vi "Scalar SV Count - type code Array.vi"(8 "Error In":errorcluster) -> (0 "Error Out":errorcluster)   [LabVIEW 2014]
doc: "This VI counts the number of scalar shared variables."
panel:
  in  "Type code Array":i32[](array[numeric])
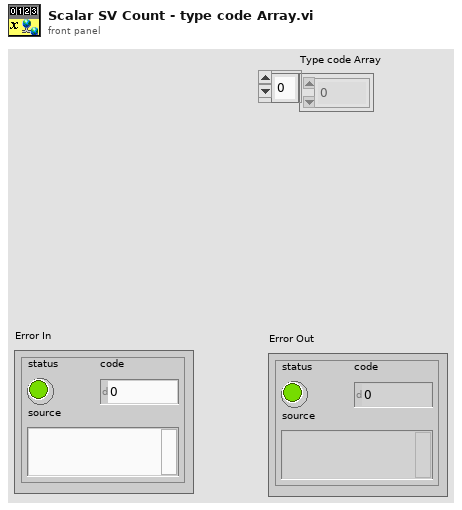
[diagram p1: front panel]
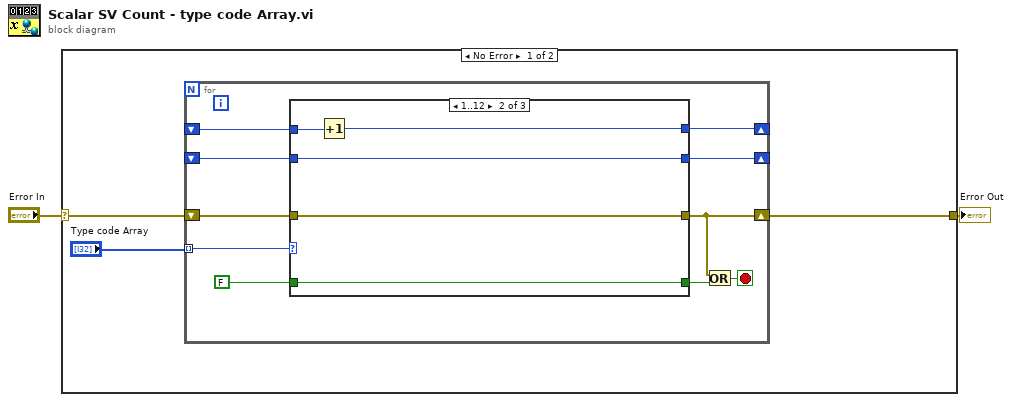
[diagram p0: block diagram]
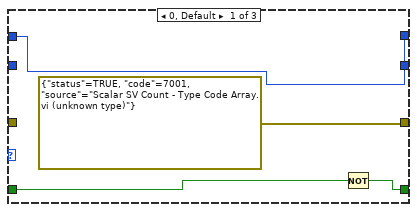
[diagram p2: hidden frame]
diagram:
  n1 = case shown="No Error" "Error In" {
    selector: "Error In" -> [w7 w30]
    tunnel: [w6 w30] -> w1
    frame No Error {
      n2 = for {
        shift-right: [w13] -> w6
        shift-left: w7 -> [w15]
        tunnel: "Type code Array" -> [w16] mode=indexing
        shift-right: [w10] -> _
        shift-left: [w12] -> w4
        shift-right: [w8] -> _
        shift-left: [w9] -> w3
        stop <- w14 stop-if-true
        n3 = case shown="1..12" w16 {
          tunnel: FALSE -> [w20 w23 w27]
          tunnel: w15 -> [_ w26 w29]
          tunnel: [errorcluster {"status"=TRUE, "code"=7001, "source"="Scalar SV Count - Type Code Array.vi (unknown type)"} ("error constant") w26 w29] -> w13
          tunnel: w12 -> [w18 w25 w28]
          tunnel: [w19 w23 w27] -> w11
          tunnel: [w18 w24 w28] -> w10
          tunnel: w9 -> [_ w22 _]
          tunnel: [_ w22 _] -> w8
          frame 0, Default {
            n4 = Not(x=w20) -> (.not. x?=w19:bool)
          }
          frame 1..12 {
            n5 = Increment(x=w25) -> (x+1=w24:u32)
          }
          frame 13..36 {
          }
        }
        n6 = Or(x=w13, y=w11) -> (x .or. y?=w14:bool)
      }
    }
    frame Error {
    }
  }
  "Error Out" <- w1
